vi "Read Results Raw.vi"(0 "VISA resource name":refnum<visa-resource-name>, 5 "Buffer number (1-8) (1)":i32=1 min=1 max=8, 11 "error in (no error)":errorcluster) -> (4 "VISA resource name out":refnum<visa-resource-name>, 6 "Raw Response":string, 15 "error out":errorcluster)   [LabVIEW 2016, in "eec EST 300.lvlib"]
doc: "RD n? Where n is the desired step number.\n\nRetrieves the raw string, unparsed data step result from the previously run test. Note you will not get a result until after the step has completed."
uses:
  <instrlib>/eec EST 300/eec EST 300.lvlib
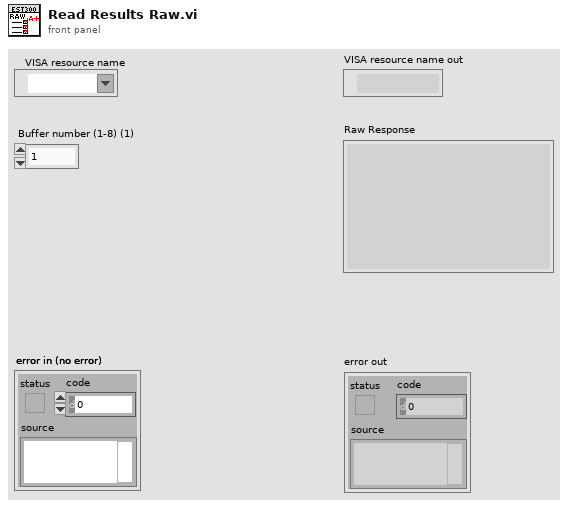
[diagram p1: front panel]
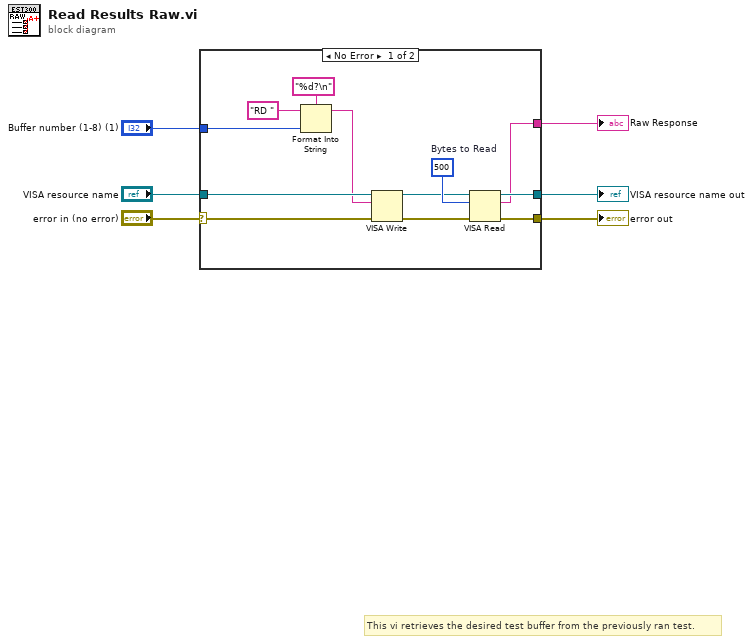
[diagram p0: block diagram]
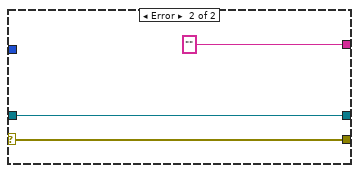
[diagram p2: hidden frame]
diagram:
  # "This vi retrieves the desired test buffer from the previously ran test."
  n1 = case shown="No Error" "error in (no error)" {
    selector: "error in (no error)" -> [w18 w21]
    tunnel: [w15 w21] -> w5
    tunnel: [w14 w20] -> w3
    tunnel: "VISA resource name" -> [w17 w20]
    tunnel: "Buffer number (1-8) (1)" -> [w16 _]
    tunnel: [w13 "" ("Decoded Response")] -> w1
    frame No Error {
      w9 = u32 500  # Bytes to Read
      n2 = Format Into String(format string="%d?\n", initial string="RD " ("string (\"\")"), w16) -> (resulting string=w10:string)  [unwired: 1 in, 1 out]
      n3 = VISA Write(VISA resource name=w17, write buffer=w10, error in (no error)=w18) -> (VISA resource name out=w7:refnum<visa-resource-name>, error out=w8:errorcluster)  [unwired: 1 out]
      n4 = VISA Read(VISA resource name=w7, byte count=w9, error in (no error)=w8) -> (VISA resource name out=w14:refnum<visa-resource-name>, read buffer=w13:string, error out=w15:errorcluster)  [unwired: 1 out]
    }
    frame Error {
    }
  }
  "error out" <- w5
  "VISA resource name out" <- w3
  "Raw Response" <- w1
